vi "DisplayValuesFromPLC_LDO.vi"(8 "error in":errorcluster, 10 "PLC Data":T1) -> (0 "error out":errorcluster, 2 "PLC Data Out":T1)   [LabVIEW 2020, in "Modbus.lvlib"]
uses:
  Modbus/Modbus.lvlib
  Modbus/Modbus PLC Data All.ctl
  Modbus/Modbus FVIR Control.ctl
  Modbus/Modbus LDO Control.ctl
  WritingDataFile/Data to Save.ctl
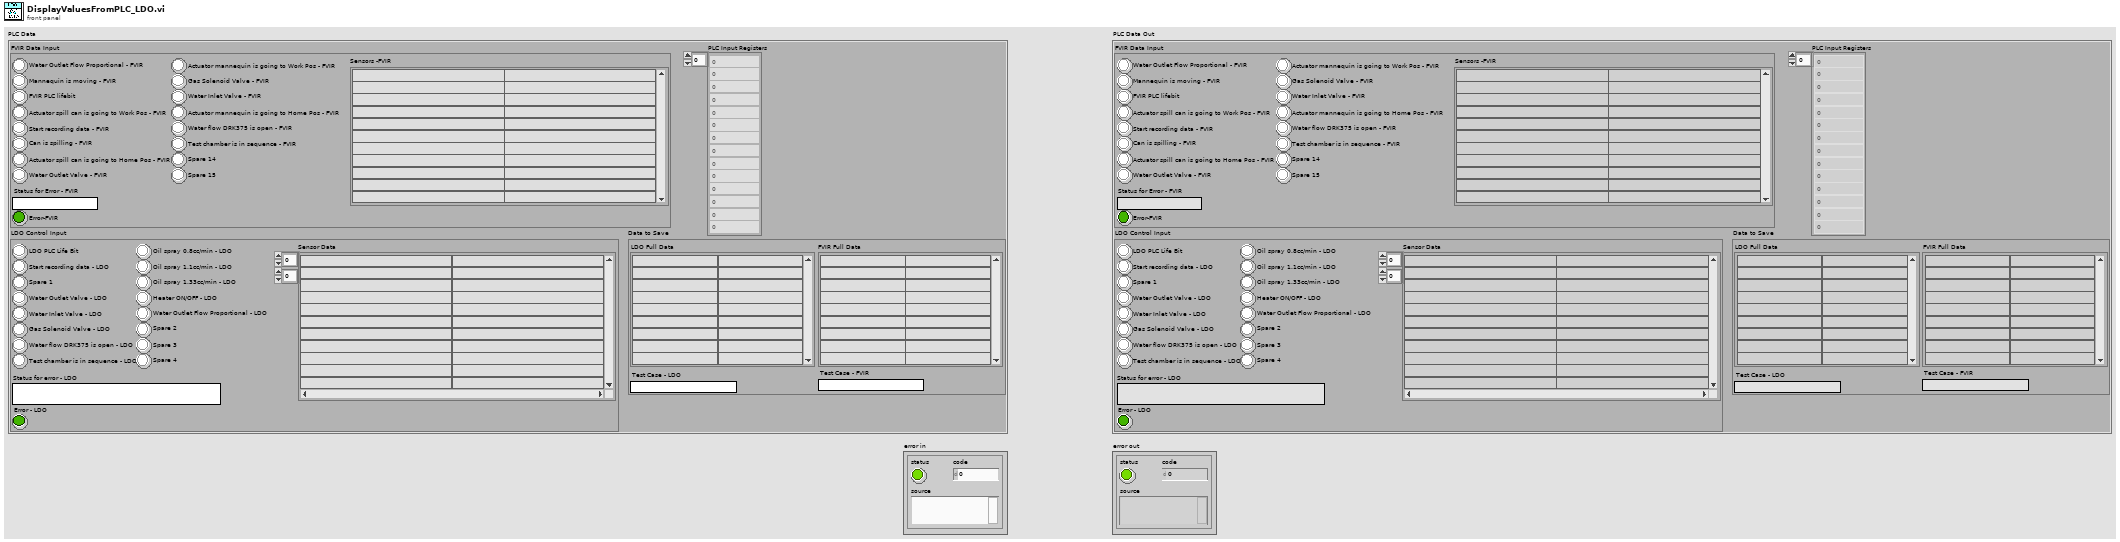
[diagram p1: front panel]
types:
  T1 = typedef "Modbus PLC Data All.ctl" = cluster{"FVIR Data Input":T2, "LDO Control Input":T3, "PLC Input Registers":u16[], "Data to Save":T4}
  T2 = typedef "Modbus FVIR Control.ctl" = cluster{"Spare 15":bool, "Spare 14":bool, "Actuator mannequin is going to Work Pos - FVIR":bool, "Actuator mannequin is going to Home Pos - FVIR":bool, "Test chamber is in sequence - FVIR ":bool, "Water flow DRK375 is open - FVIR":bool, "Gas Solenoid Valve - FVIR":bool, "Water Inlet Valve - FVIR":bool, "Water Outlet Flow Proportional - FVIR":bool, "Start recording data - FVIR":bool, "Actuator spill can is going to Work Pos - FVIR":bool, "Actuator spill can is going to Home Pos - FVIR":bool, "Water Outlet Valve - FVIR":bool, "Can is spilling - FVIR":bool, "Mannequin is moving - FVIR":bool, "FVIR PLC lifebit":bool, "Status for Error - FVIR":string, "Error-FVIR":bool, "Sensors -FVIR":string[][]}
  T3 = typedef "Modbus LDO Control.ctl" = cluster{"LDO PLC Life Bit":bool, "Start recording data - LDO":bool, "Spare 1":bool, "Water Outlet Valve - LDO":bool, "Water Inlet Valve - LDO":bool, "Gas Solenoid Valve - LDO":bool, "Water flow DRK375 is open - LDO":bool, "Test chamber is in sequence - LDO":bool, "Oil spray 0.8cc/min - LDO":bool, "Oil spray 1.1cc/min - LDO":bool, "Oil spray 1.33cc/min - LDO":bool, "Heater ON/OFF - LDO":bool, "Water Outlet Flow Proportional - LDO":bool, "Spare 2":bool, "Spare 3":bool, "Spare 4":bool, "Status for error - LDO":string, "Error - LDO":bool, "Sensor Data":string[][]}
  T4 = typedef "Data to Save.ctl" = cluster{"LDO Full Data":string[][], "FVIR Full Data":string[][], "Test Case - FVIR":string, "Test Case - LDO":string}
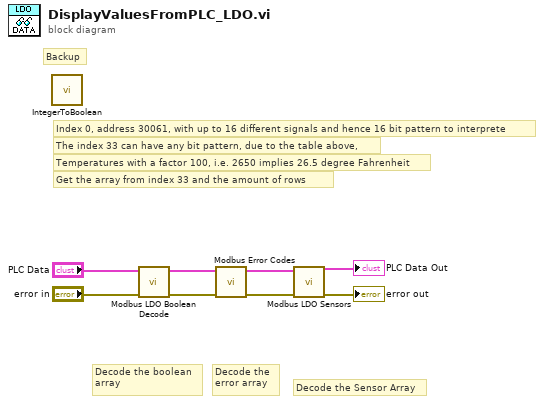
[diagram p0: block diagram]
diagram:
  # "Decode the Sensor Array"
  # "Decode the \nerror array"
  # "Decode the boolean\narray"
  # "Index 0, address 30061, with up to 16 different signals and hence 16 bit pattern to interprete"
  # "The index 33 can have any bit pattern, due to the table above,"
  # "Backup"
  # "Get the array from index 33 and the amount of rows"
  # "Temperatures with a factor 100, i.e. 2650 implies 26.5 degree Fahrenheit"
  n1 = call "IntegerToBoolean.vi"() -> ()  [unwired: 11 in, 1 out]
  n2 = call "Modbus LDO Boolean Decode.vi"("error in"="error in", "PLC Data"="PLC Data") -> ("error out"=w7:errorcluster, "PLC Data Out"=w3:T1)  [unwired: 8 in]
  n3 = call "Modbus Error Codes.vi"("error in"=w7, "PLC Data"=w3) -> ("error out"=w8:errorcluster, "PLC Data Output"=w2:T1)  [unwired: 8 in]
  n4 = call "Modbus LDO Sensors.vi"("error in"=w8, "PLC Data"=w2) -> ("error out"=→"error out":errorcluster, "PLC Data Output"=→"PLC Data Out":T1)  [unwired: 8 in]
